vi "Lights Controller.vi"(0 "Lights 1":bool, 1 "Light Period":dbl, 5 "Lights 2":bool, 7 "Turn Signal":i8(slide) scale=-1.0..1.0, 9 "Break":bool, 11 "Lights Flag":bool, 12 "Under Lights":bool, 13 "Start Engine":bool) -> (2 "Blue Duty":dbl, 3 "Light Period Out":dbl, 4 "Red  Duty":dbl, 6 "White Duty":dbl, 8 "Orange L Duty":dbl, 10 "Orange R Duty":dbl, 15 "Lights Flag Out":bool)   [LabVIEW 2015]
panel:
  # "Left"
  # "Right"
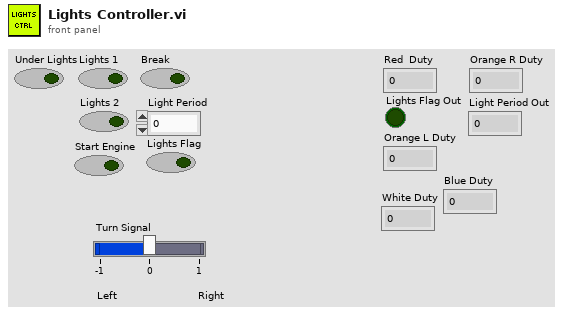
[diagram p1: front panel]
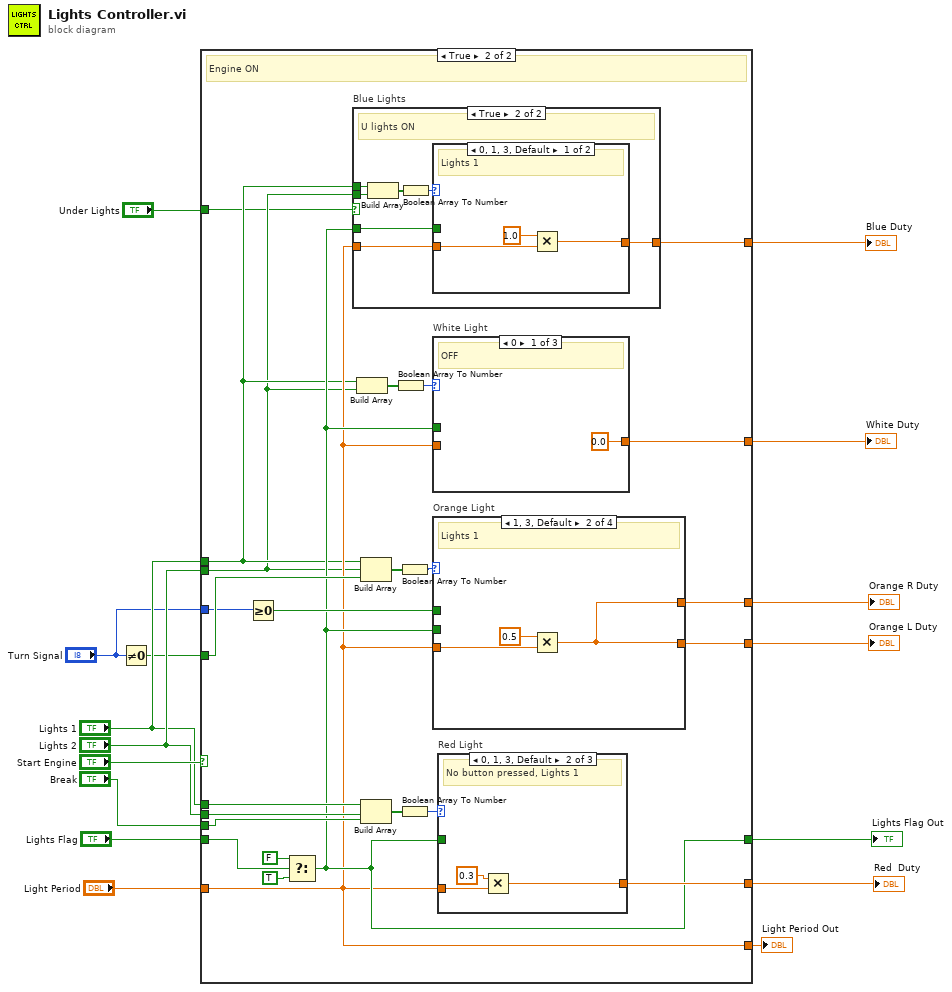
[diagram p0: block diagram]
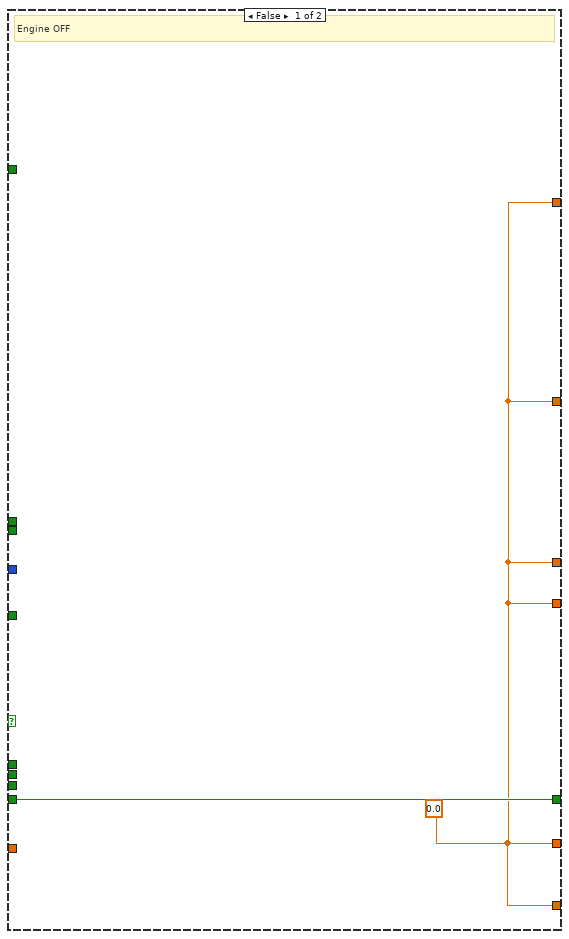
[diagram p2: hidden frame]
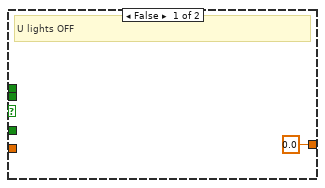
[diagram p3: hidden frame]
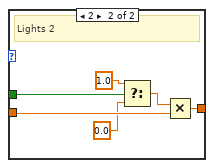
[diagram p4: hidden frame]
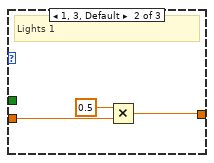
[diagram p5: hidden frame]
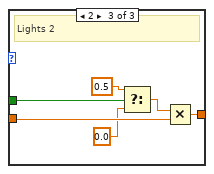
[diagram p6: hidden frame]
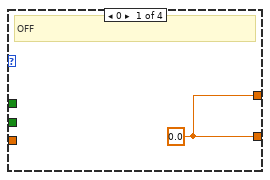
[diagram p7: hidden frame]
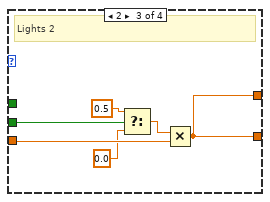
[diagram p8: hidden frame]
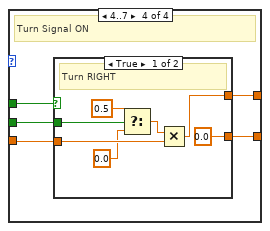
[diagram p9: hidden frame]
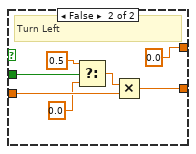
[diagram p10: hidden frame]
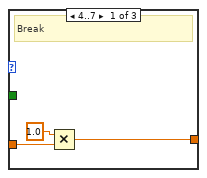
[diagram p11: hidden frame]
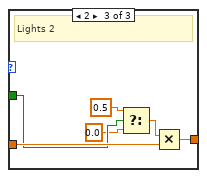
[diagram p12: hidden frame]
diagram:
  n1 = Not Equal To 0?(x="Turn Signal") -> (x != 0?=w5:bool)
  n2 = case shown="True" "Start Engine" {
    tunnel: "Lights 2" -> [_ w30]
    tunnel: "Lights 1" -> [_ w29]
    tunnel: "Break" -> [_ w40]
    tunnel: "Light Period" -> [_ w23]
    tunnel: [w17 w41] -> w11
    tunnel: "Lights Flag" -> [w18 w34]
    tunnel: [w18 w24] -> w12
    tunnel: "Lights 2" -> [_ w21]
    tunnel: "Lights 1" -> [_ w22]
    tunnel: [w17 w37] -> w8
    tunnel: [w17 w31] -> w7
    tunnel: [w17 w28] -> w6
    tunnel: w5 -> [_ w27]
    tunnel: "Turn Signal" -> [_ w26]
    tunnel: [w17 w23] -> w3
    tunnel: "Under Lights" -> [_ w20]
    tunnel: [w17 w19] -> w1
    frame False {
      w17 = 0.0
      # "Engine OFF"
    }
    frame True {
      # "Engine ON"
      n3 = Greater Or Equal To 0?(x=w26) -> (x >= 0?=w25:bool)
      n4 = Select(t=FALSE ("Lights Flag"), s=w34, f=TRUE ("Lights Flag")) -> (s? t:f=w24:bool)
      n5 = case "Blue Lights" shown="True" w20 {
        tunnel: w24 -> [_ w49]
        tunnel: w23 -> [_ w48]
        tunnel: w22 -> [_ w47]
        tunnel: w21 -> [_ w46]
        tunnel: [0.0 ("x") w45] -> w19
        frame False {
          # "U lights OFF"
        }
        frame True {
          # "U lights ON"
          n6 = Build Array(w47, w46) -> (w50:bool[])
          n7 = Boolean Array To Number(Boolean array=w50) -> (number=w51:u32)
          n8 = case "Blue Light" shown="0, 1, 3, Default" w51 {
            tunnel: [w54 w60] -> w45
            tunnel: w48 -> [w53 w57]
            tunnel: w49 -> [_ w56]
            frame 0, 1, 3, Default {
              # "Lights 1"
              n9 = Multiply(x=1.0, y=w53) -> (x*y=w54:dbl)
            }
            frame 2 {
              # "Lights 2"
              n10 = Select(t=1.0 ("x"), s=w56, f=0.0 ("x")) -> (s? t:f=w58:dbl)
              n11 = Multiply(x=w58, y=w57) -> (x*y=w60:dbl)
            }
          }
        }
      }
      n12 = Build Array(w22, w21) -> (w33:bool[])
      n13 = Build Array(w22, w21, w27) -> (w39:bool[])
      n14 = Build Array(w29, w30, w40) -> (w43:bool[])
      n15 = Boolean Array To Number(Boolean array=w33) -> (number=w32:u32)
      n16 = Boolean Array To Number(Boolean array=w39) -> (number=w38:u32)
      n17 = Boolean Array To Number(Boolean array=w43) -> (number=w42:u32)
      n18 = case "White Light" shown="0" w32 {
        tunnel: [0.0 ("x") w64 w70] -> w31
        tunnel: w23 -> [_ w63 w67]
        tunnel: w24 -> [_ _ w66]
        frame 0 {
          # "OFF"
        }
        frame 1, 3, Default {
          # "Lights 1"
          n19 = Multiply(x=0.5, y=w63) -> (x*y=w64:dbl)
        }
        frame 2 {
          # "Lights 2"
          n20 = Select(t=0.5 ("x"), s=w66, f=0.0 ("x")) -> (s? t:f=w68:dbl)
          n21 = Multiply(x=w68, y=w67) -> (x*y=w70:dbl)
        }
      }
      n22 = case "Orange Light" shown="1, 3, Default" w38 {
        tunnel: [w71 w72 w75 w82] -> w37
        tunnel: w23 -> [_ w74 w78 w85]
        tunnel: w24 -> [_ _ w77 w84]
        tunnel: [w71 w72 w75 w83] -> w28
        tunnel: w25 -> [_ _ _ w81]
        frame 0 {
          w71 = 0.0 ("x")
          # "OFF"
        }
        frame 1, 3, Default {
          # "Lights 1"
          n23 = Multiply(x=0.5, y=w74) -> (x*y=w72:dbl)
        }
        frame 2 {
          # "Lights 2"
          n24 = Select(t=0.5 ("x"), s=w77, f=0.0 ("x")) -> (s? t:f=w79:dbl)
          n25 = Multiply(x=w79, y=w78) -> (x*y=w75:dbl)
        }
        frame 4..7 {
          # "Turn Signal ON"
          n26 = case shown="True" w81 {
            tunnel: w85 -> [w90 w97]
            tunnel: w84 -> [w89 w96]
            tunnel: [w87 0.0 ("x")] -> w83
            tunnel: [0.0 ("x") w93] -> w82
            frame True {
              # "Turn RIGHT"
              n27 = Select(t=0.5 ("x"), s=w89, f=0.0 ("x")) -> (s? t:f=w91:dbl)
              n28 = Multiply(x=w91, y=w90) -> (x*y=w87:dbl)
            }
            frame False {
              # "Turn Left"
              n29 = Select(t=0.5 ("x"), s=w96, f=0.0 ("x")) -> (s? t:f=w98:dbl)
              n30 = Multiply(x=w98, y=w97) -> (x*y=w93:dbl)
            }
          }
        }
      }
      n31 = case "Red Light" shown="0, 1, 3, Default" w42 {
        tunnel: w23 -> [w102 w105 w111]
        tunnel: [w100 w103 w110] -> w41
        tunnel: w24 -> [_ _ w109]
        frame 4..7 {
          # "Break"
          n32 = Multiply(x=1.0, y=w102) -> (x*y=w100:dbl)
        }
        frame 0, 1, 3, Default {
          # "No button pressed, Lights 1"
          n33 = Multiply(x=0.3, y=w105) -> (x*y=w103:dbl)
        }
        frame 2 {
          # "Lights 2"
          n34 = Select(t=0.5 ("x"), s=w109, f=0.0 ("x")) -> (s? t:f=w106:dbl)
          n35 = Multiply(x=w106, y=w111) -> (x*y=w110:dbl)
        }
      }
    }
  }
  "Red  Duty" <- w11
  "Lights Flag Out" <- w12
  "Orange L Duty" <- w8
  "White Duty" <- w7
  "Orange R Duty" <- w6
  "Light Period Out" <- w3
  "Blue Duty" <- w1
